vi "group Bulk Write Add Param.vi"(5 "input_length":u16, 6 "data":u32, 7 "data_length":u16, 9 "start_address":u16, 10 "id":u8, 11 "group_num":i32) -> (3 "function return":u8)   [LabVIEW 2015, in "dxl_x86_c.lvlib"]
doc: "WINDECLSPEC uint8_t groupBulkWriteAddParam (int group_num, uint8_t id, uint16_t start_address, uint16_t data_length, uint32_t data, uint16_t input_length);"
uses:
  dxl_x86_c.lvlib
  dxl_x86_c.dll
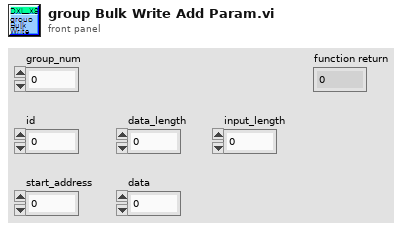
[diagram p1: front panel]
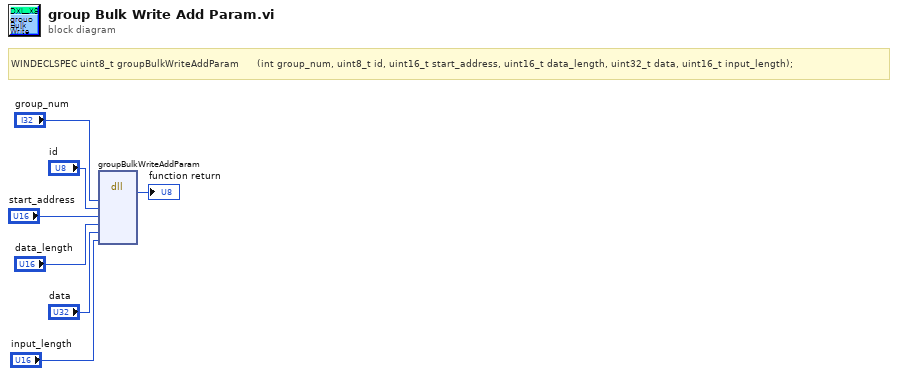
[diagram p0: block diagram]
diagram:
  # "WINDECLSPEC uint8_t groupBulkWriteAddParam      (int group_num, uint8_t id, uint16_t start_address, uint16_t data_length, uint32_t data, uint16_t input_length);"
  n1 = dll-call lib="C:/Users/Platform/Desktop/LabVIEW/dxl_x86_c.lvlib/dxl_x86_c.*" fn="groupBulkWriteAddParam"("group_num"="group_num", "id"="id", "start_address"="start_address", "data_length"="data_length", "data"="data", "input_length"="input_length") -> (→"function return":u8)  [unwired: 9 in, 2 out]
